vi "View.vi"() -> ()   [LabVIEW 2020, in "simple_html_chat_ui.lvclass"]
uses:
  simple_html_chat_ui.lvclass
  D:/Personal/LabVIEW LLMs/user_interfaces/simple_html_chat_ui/assembly_support/Microsoft.Web.WebView2.WinForms.dll
  assembly_support/Microsoft.Web.WebView2.WinForms.dll
  typedefs/ui_user_event.ctl
  D:/Personal/LabVIEW LLMs/user_interfaces/simple_html_chat_ui/assembly_support/Microsoft.Web.WebView2.Core.dll
  assembly_support/Microsoft.Web.WebView2.Core.dll
panel:
  in  "WebView2":refnum<k24>(container)
  out "error out":errorcluster
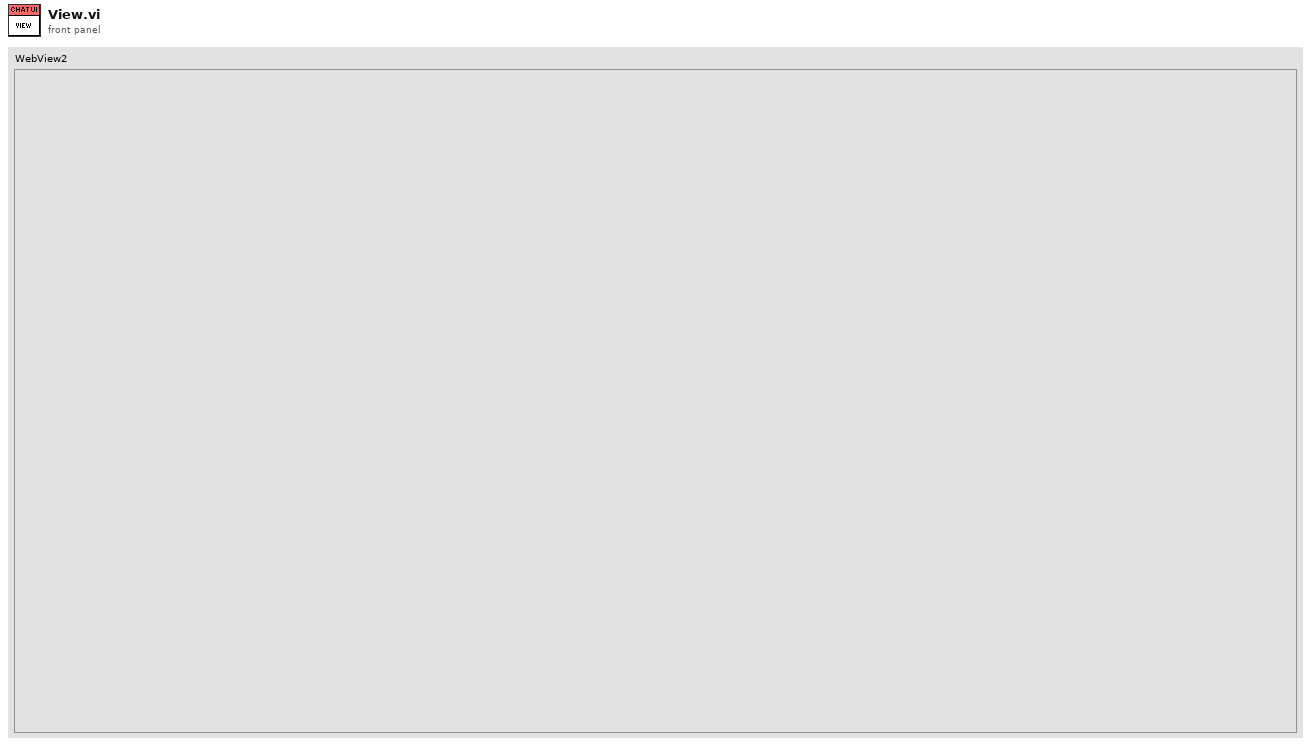
[diagram p1: front panel]
types:
  T1 = typedef "simple_html_chat_ui.lvclass/ui_user_event.ctl" = enum16{"Initialize", "Generate", "Get Reference", "Destroy"}
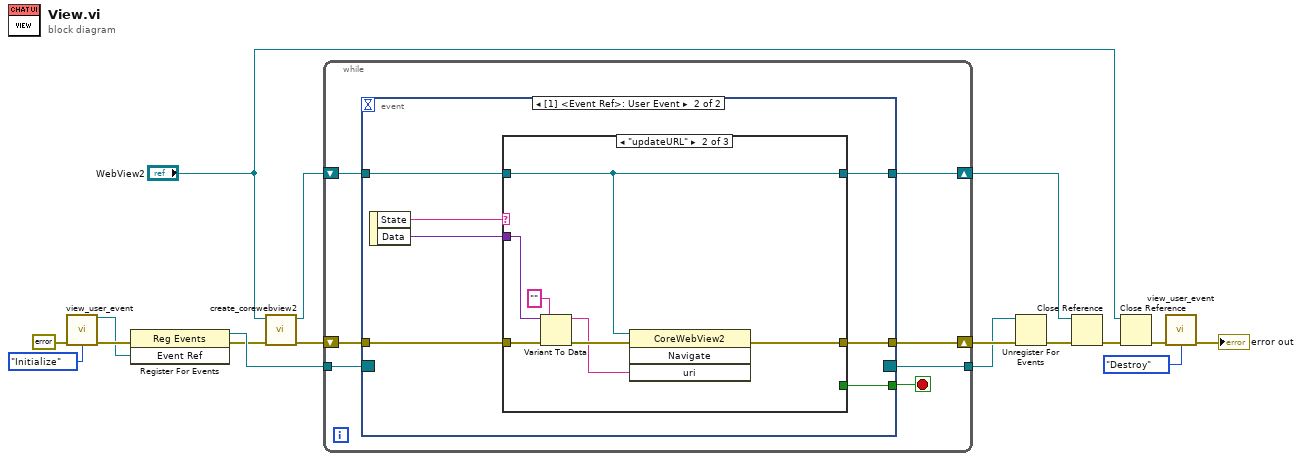
[diagram p0: block diagram]
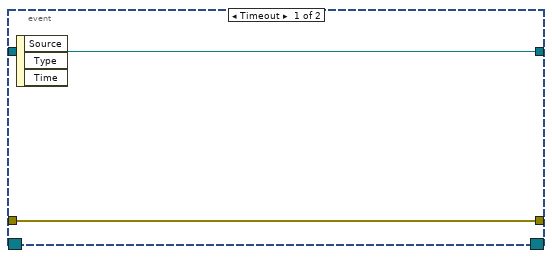
[diagram p2: hidden frame]
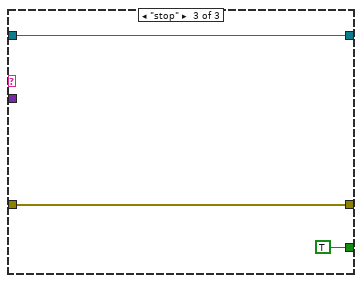
[diagram p4: hidden frame]
diagram:
  n1 = call "view_user_event.vi"("error in (no error)"=errorcluster {"status"=FALSE, "code"=0, "source"=""}, "Operation"=ui_user_event."Initialize") -> ("Event Ref"=w14:refnum<user-event>, "error out"=w15:errorcluster)  [unwired: 12 in]
  n2 = register-events(error in=w15, w14) -> (reference out=w13:refnum<event-registration>, error out=w6:errorcluster)  [unwired: 1 in]
  n3 = call "create_corewebview2.vi"("error in"=w6, "WebView2"="WebView2") -> ("error out"=w5:errorcluster, "CoreWebView2"=w4:refnum<k24>)  [unwired: 8 in]
  n4 = while {
    shift-right: [w20] -> w12
    shift-left: w5 -> [w23]
    tunnel: w13 -> [w24]
    shift-right: [w21] -> w9
    shift-left: w4 -> [w22]
    tunnel: [w18] -> w11
    stop <- w19 stop-if-true
    n5 = event shown="[1] <Event Ref>: User Event" {
      selector: w24 -> [_ _]
      dyn-events: [_ _] -> w18
      timeout: _ -> [_ _]
      tunnel: w23 -> [w25 w32]
      tunnel: w22 -> [w26 w31]
      tunnel: [w26 w30] -> w21
      tunnel: [w25 w28] -> w20
      tunnel: [_ w27] -> w19
      event Timeout {
        n6 = event-data() -> ()  [unwired: 1 in, 3 out]
      }
      event User Event {
        n7 = event-data() -> ("State"=w33:string, "Data"=w29:variant)  [unwired: 1 in]
        n8 = case shown="\"updateURL\"" w33 {
          tunnel: w32 -> [w34 w40 w44]
          tunnel: w31 -> [w35 w42 w45]
          tunnel: [w35 w42 w45] -> w30
          tunnel: w29 -> [_ w39 _]
          tunnel: [w34 w36 w44] -> w28
          tunnel: [_ _ TRUE] -> w27
          frame Default {
          }
          frame "updateURL" {
            n9 = Variant To Data(error in=w40, type="", Variant=w39) -> (data=w37:string, error out=w41:errorcluster)
            n10 = invoke class="CoreWebView2" method="Navigate"(reference=w42, error in=w41, "uri"=w37) -> (error out=w36:errorcluster)  [unwired: 1 in, 3 out]
          }
          frame "stop" {
          }
        }
      }
    }
  }
  n11 = Unregister For Events(event registration refnum=w11, error in=w12) -> (error out=w10:errorcluster)
  n12 = Close Reference(reference=w9, error in (no error)=w10) -> (error out=w3:errorcluster)
  n13 = Close Reference(reference="WebView2", error in (no error)=w3) -> (error out=w2:errorcluster)
  n14 = call "view_user_event.vi"("error in (no error)"=w2, "Operation"=ui_user_event."Destroy") -> ("error out"=→"error out":errorcluster)  [unwired: 12 in, 1 out]
